vi "WVDIAL_Main.vi"() -> ()   [LabVIEW 2012]
uses:
  WVDIAL_GlobalVariables.vi
  TypeDefinitions.llb/TypeDef_LoopStagesMain.ctl
  TypeDefinitions.llb/TypeDef_ConfigureFIleTypes.ctl
  TypeDefinitions.llb/TypeDef_MainControlSystem.ctl
  TypeDefinitions.llb/TypeDef_ChildResponding.ctl
panel:
  out "Children Responding":T1[](array[typedef])
  out "LoopCounter":i32
  out "Permission Level":T3(ring)
  in  "User Comment":bool
  in  "Update Permissions":bool
  in  "Global Abort":bool
  in  "Tab Control":T4(tab)
  in  "Software Testing":bool
  in  "Template":bool
  in  "Operations":bool
  in  "Warmup":bool
  out "error IO":errorcluster
  out "SubPanelWidth":i32
  out "SubPanelHeight":i32
  out "What to Do":string
  out "QueueElement":string
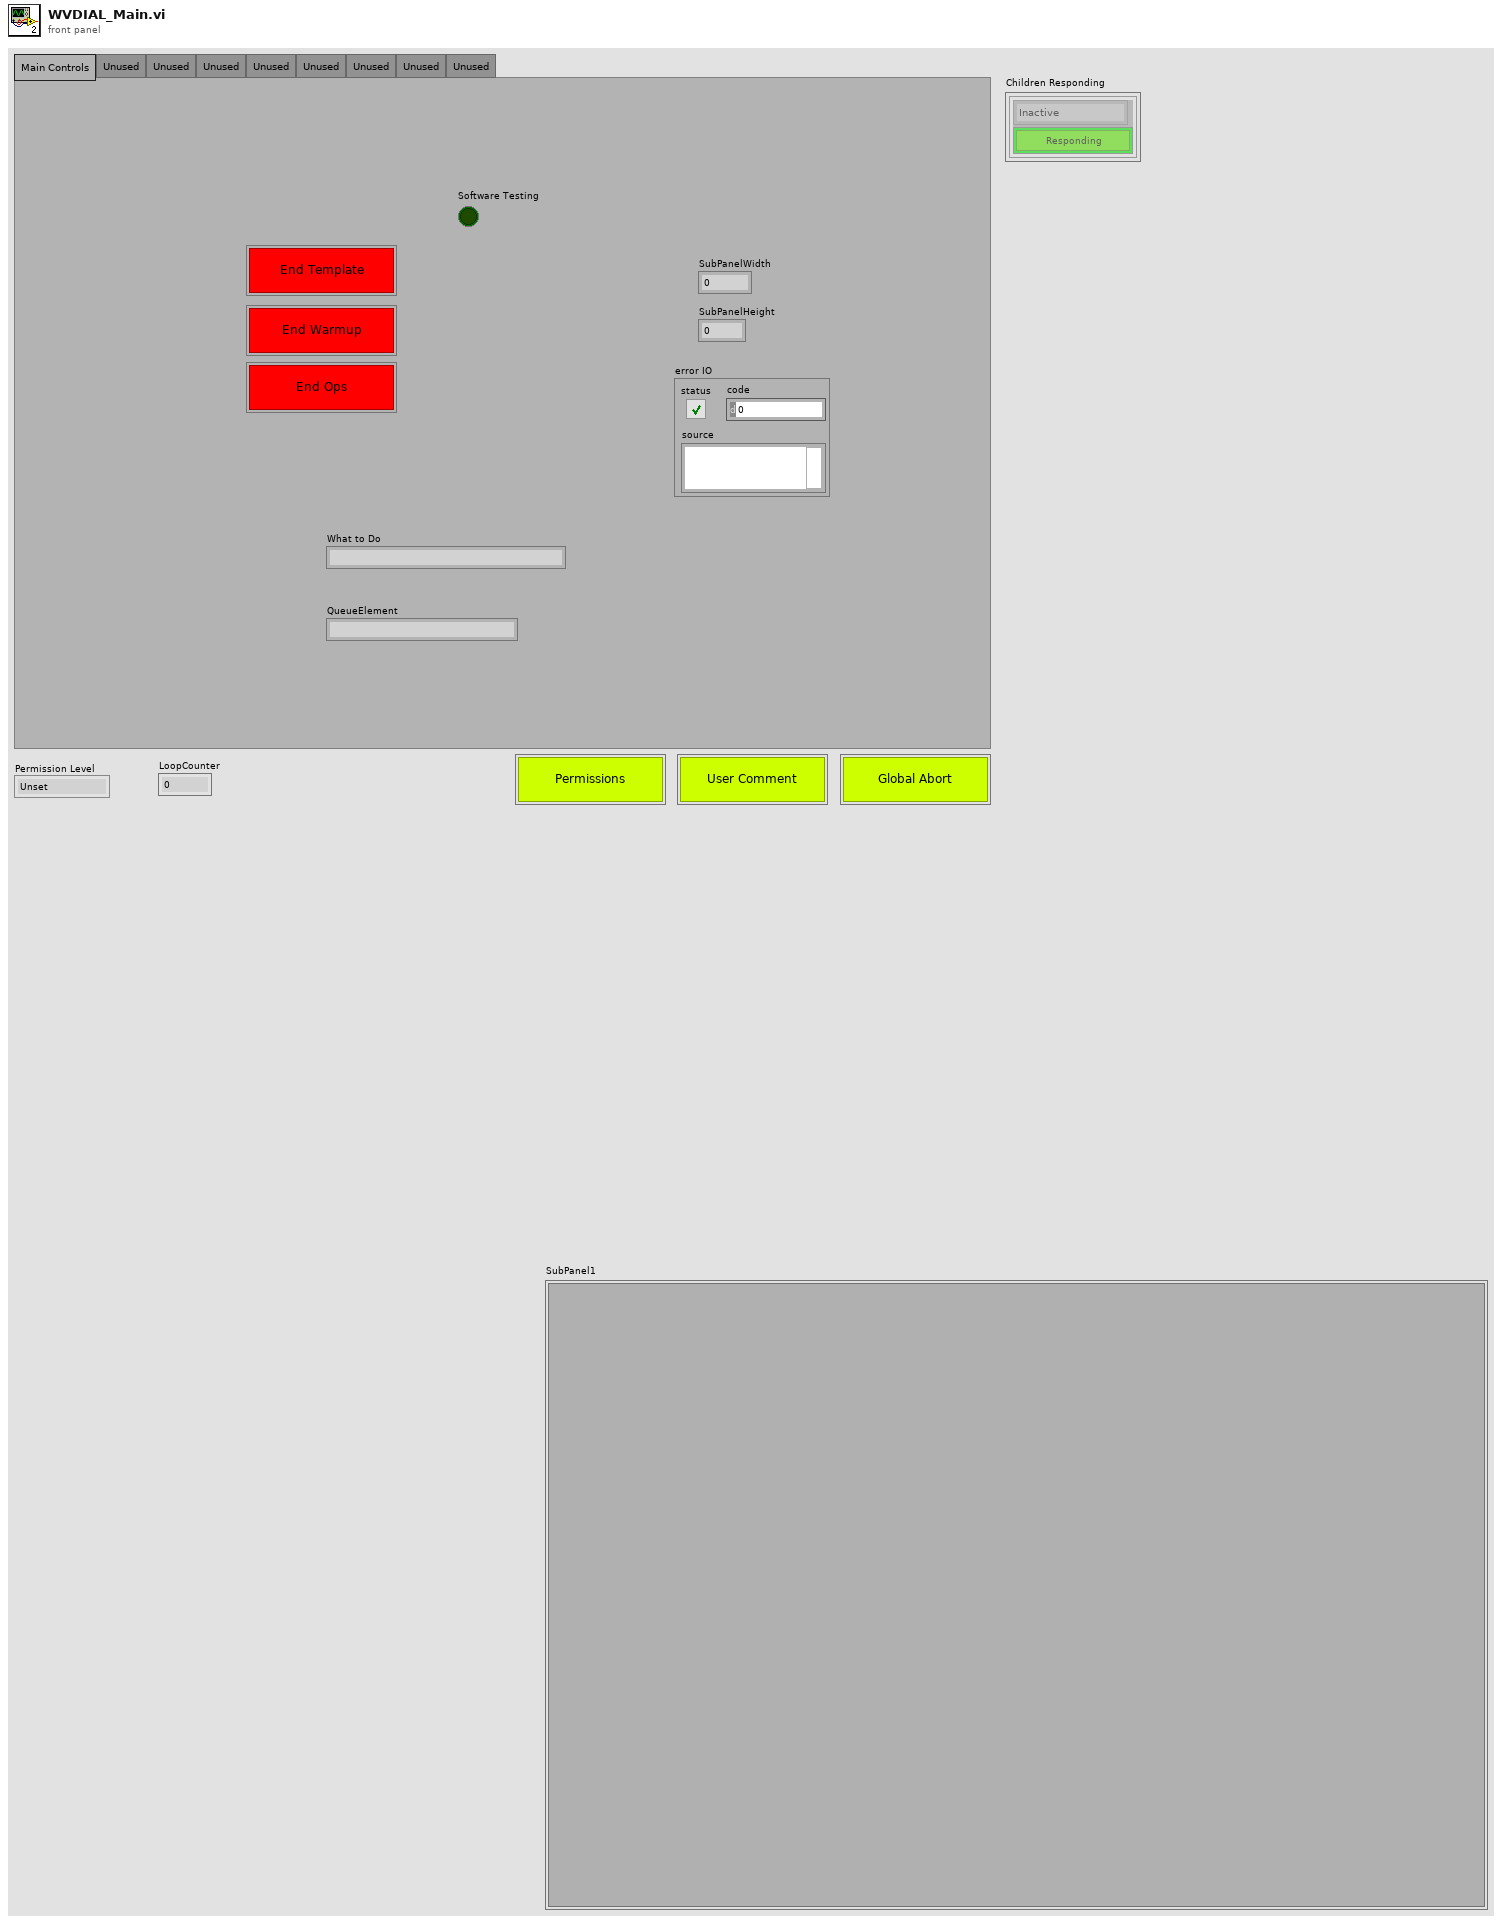
[diagram p1: front panel]
types:
  T1 = typedef "TypeDef_ChildResponding.ctl" = cluster{"MainControlSystems":T2, "Responding":bool}
  T2 = typedef "TypeDef_MainControlSystem.ctl" = enum16{"Inactive", "MCSControl", "MCSDisplay", "LaserControl", "LaserLocking", "WeatherStation", "DataDisplay", "Template"}
  T3 = enum16{"Unset", "Operator", "Administrator", "Full"}
  T4 = enum32{"Main Controls", "Inner Function 1", "Inner Function 2", "Inner Function 3", "Inner Function 4", "Inner Function 5", "Inner Function 6", "Inner Function 7", "Inner Function 8"}
  T5 = typedef "TypeDef_LoopStagesMain.ctl" = enum16{"Configure", "Initialize", "Idle", "ExitChildren", "Error Handler", "Exit"}
  T6 = typedef "TypeDef_ConfigureFIleTypes.ctl" = enum16{"Main", "OpsMain", "OpsTemplate", "OpsWarmup", "ChildHousekeeping", "ChildLaserLocking", "ChildMCS", "ChildMCSControl", "ChildPowerSwitches", "ChildQuantumComposer", "ChildTemplate", "ChildUPS", "ChildWeatherStation", "ChildPlotting", "TestingSwitches", "TestingWavemeter"}
  T7 = cluster{"MainControlSystems":T2, "Responding":bool}[]
  T8 = cluster{"Child Command Stop":bool, "Child Responding":bool, "MainControlSystems":T2, "LastReportTime":dbl, "Child Exiting":bool}[]
  T9 = enum32{"Page Enabled", "Page Disabled", "Page Disabled & Grayed"}
  T10 = cluster{"Child Command Stop":bool, "Child Responding":bool, "MainControlSystems":T2, "LastReportTime":dbl, "Child Exiting":bool}
  T11 = typedef "TypeDef_ChildReporting.ctl" = cluster{"Child Command Stop":bool, "Child Responding":bool, "MainControlSystems":T2, "LastReportTime":dbl, "Child Exiting":bool}
  T12 = enum32{"Bad", "Idle", "Run top level", "Running"}
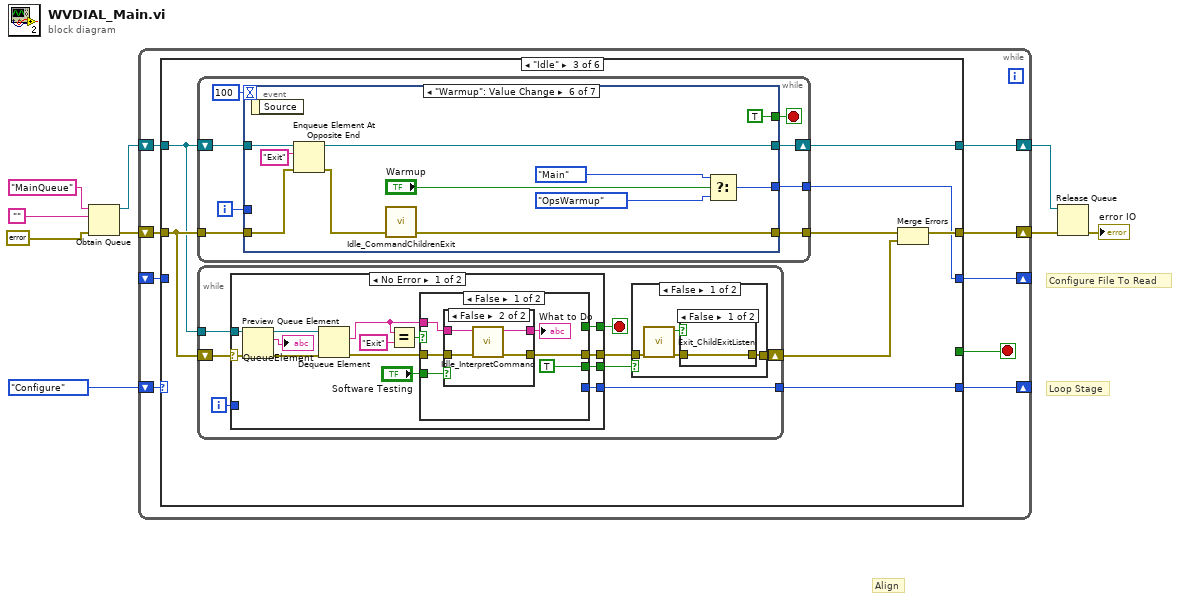
[diagram p0: block diagram]
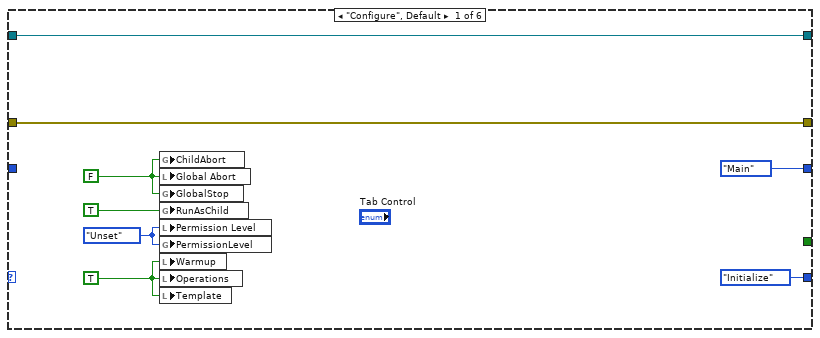
[diagram p2: hidden frame]
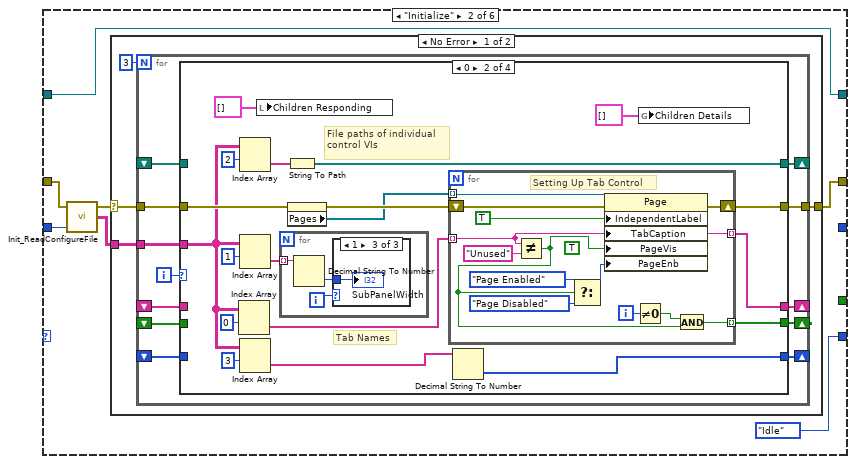
[diagram p3: hidden frame]
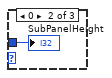
[diagram p6: hidden frame]
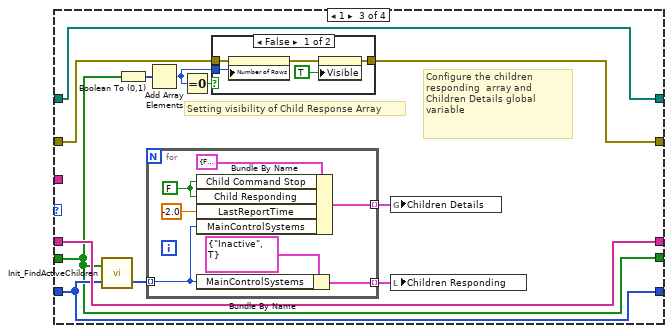
[diagram p7: hidden frame]
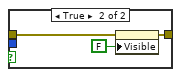
[diagram p8: hidden frame]
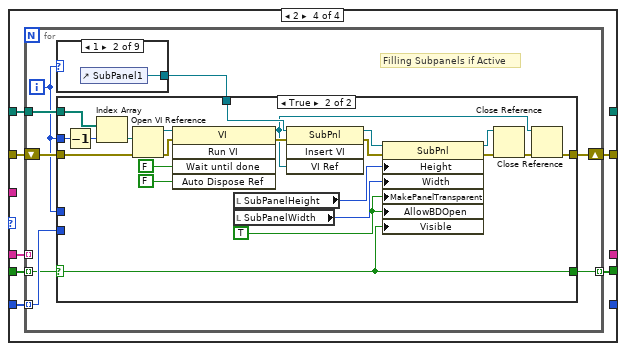
[diagram p9: hidden frame]
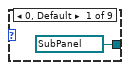
[diagram p11: hidden frame]
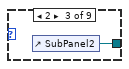
[diagram p12: hidden frame]
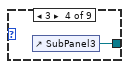
[diagram p13: hidden frame]
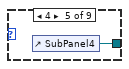
[diagram p14: hidden frame]
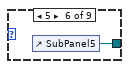
[diagram p15: hidden frame]
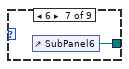
[diagram p16: hidden frame]
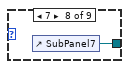
[diagram p17: hidden frame]
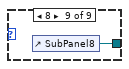
[diagram p18: hidden frame]
diagram:
  # "Align"
  # "Configure File To Read"
  # "Loop Stage"
  n1 = Obtain Queue(name (unnamed)="MainQueue", element data type="", error in (no error)=errorcluster {"status"=FALSE, "code"=0, "source"=""}) -> (queue out=w2:refnum<queue>, error out=w3:errorcluster)  [unwired: 2 in, 1 out]
  n2 = while {
    shift-right: [w14] -> w7
    shift-left: w3 -> [w15]
    shift-right: [w13] -> w8
    shift-left: w2 -> [w12]
    shift-right: [w17] -> _
    shift-left: TypeDef_LoopStagesMain."Configure" ("Enum") -> [w18]
    shift-right: [w11] -> _
    shift-left: _ -> [w10]
    stop <- w16 stop-if-true
    n3 = case shown="\"Idle\"" w18 {
      tunnel: [TypeDef_LoopStagesMain."Initialize" ("Enum") TypeDef_LoopStagesMain."Idle" ("Enum") w173 TypeDef_LoopStagesMain."Initialize" ("Enum") TypeDef_LoopStagesMain."Idle" ("Enum") TypeDef_LoopStagesMain."Exit" ("Enum")] -> w17
      tunnel: [_ _ _ _ _ TRUE] -> w16
      tunnel: [w23 w32 w170 w290 w319 w321] -> w14
      tunnel: w15 -> [w23 w30 w174 w291 w319 w325]
      tunnel: [w24 w31 w175 w294 w317 w327] -> w13
      tunnel: w12 -> [w24 w31 w169 w294 w317 w327]
      tunnel: [TypeDef_ConfigureFIleTypes."Main" ("MainControlSystems") _ w168 w292 _ _] -> w11
      tunnel: w10 -> [_ w27 _ w292 _ _]
      frame "Configure", Default {
        w20 = TRUE ("Warmup")
        w19 = T3."Unset" ("Permission Level")
        w21 = FALSE ("Global Stop")
        n4 = global write "WVDIAL_GlobalVariables.vi" "ChildAbort"(w21) -> ()
        n5 = local write "Global Abort"(w21) -> ()
        n6 = global write "WVDIAL_GlobalVariables.vi" "GlobalStop"(w21) -> ()
        n7 = global write "WVDIAL_GlobalVariables.vi" "RunAsChild"(TRUE ("RunAsChild")) -> ()
        n8 = local write "Permission Level"(w19) -> ()
        n9 = global write "WVDIAL_GlobalVariables.vi" "PermissionLevel"(w19) -> ()
        n10 = local write "Warmup"(w20) -> ()
        n11 = local write "Operations"(w20) -> ()
        n12 = local write "Template"(w20) -> ()
      }
      frame "Initialize" {
        n13 = call "Init_ReadConfigureFile.vi"("ConfigureFileType"=w27, "error in"=w30) -> ("Parsed List"=w28:string[][], "error out"=w29:errorcluster)  [unwired: 1 in, 1 out]
        n14 = case shown="No Error" w29 {
          selector: w29 -> [w36 w167]
          tunnel: [w37 w167] -> w32
          tunnel: w28 -> [w35 _]
          frame No Error {
            n15 = for {
              N: 3 -> [_]
              tunnel: [w49] -> w37
              tunnel: w36 -> [w40]
              tunnel: w35 -> [w47]
              shift-right: [w46] -> _
              shift-left: _ -> [w45]
              shift-right: [w44] -> _
              shift-left: _ -> [w43]
              shift-right: [w42] -> _
              shift-left: _ -> [w41]
              shift-right: [w39] -> _
              shift-left: _ -> [w38]
              i -> [w48]
              n16 = case shown="0" w48 {
                tunnel: [w53 w64 w100 w125] -> w49
                tunnel: w40 -> [w53 w63 w101 w121]
                tunnel: w47 -> [_ w59 _ _]
                tunnel: [w54 w69 w93 _] -> w46
                tunnel: w45 -> [w54 _ w93 w124]
                tunnel: [w52 w66 w97 _] -> w44
                tunnel: w43 -> [w52 _ w97 w123]
                tunnel: [w51 w65 w95 w120] -> w42
                tunnel: w41 -> [w51 _ w95 w122]
                tunnel: [w50 w57 w96 _] -> w39
                tunnel: w38 -> [w50 _ w96 w119]
                frame -1, Default {
                }
                frame 0 {
                  # "File paths of individual control VIs"
                  # "Tab Names"
                  n17 = Index Array(array=w59, index (row)=0) -> (element=w67:string[])  [unwired: 1 in]
                  n18 = Index Array(array=w59, index (row)=2) -> (element=w70:string[])  [unwired: 1 in]
                  n19 = Index Array(array=w59, index (row)=1) -> (element=w68:string[])  [unwired: 1 in]
                  n20 = Index Array(array=w59, index (row)=3) -> (element=w58:string[])  [unwired: 1 in]
                  n21 = local write "Children Responding"(T7 [] ("Children Responding")) -> ()
                  n22 = for {
                    tunnel: w68 -> [w88] mode=indexing
                    i -> [w89]
                    n23 = Decimal String To Number(string=w88) -> (number=w87:i32)  [unwired: 2 in, 1 out]
                    n24 = case shown="1" w89 {
                      tunnel: w87 -> [_ w90 w91]
                      frame -1, Default {
                      }
                      frame 0 {
                        "SubPanelHeight" <- w90
                      }
                      frame 1 {
                        "SubPanelWidth" <- w91
                      }
                    }
                  }
                  n25 = String To Path(string=w70) -> (path=w69:path[])
                  n26 = property on="Tab Control" class="TabCtl (strict)"(error in=w63) -> (error out=w62:errorcluster, "Pages"=w61:refnum<vi>[])  [unwired: 1 in, 1 out]
                  n27 = for {
                    tunnel: w67 -> [w80] mode=indexing
                    tunnel: w61 -> [w83] mode=indexing
                    shift-right: [w81] -> w64
                    shift-left: w62 -> [w82]
                    tunnel: [w80] -> w66 mode=indexing
                    tunnel: [w77] -> w65 mode=indexing
                    i -> [w78]
                    (unwired) TRUE ("Page Visible")
                    # "Setting Up Tab Control"
                    n28 = Not Equal?(x=w80, y="Unused") -> (x != y?=w76:bool)
                    n29 = Select(t=T9."Page Enabled" ("Page Enabled State"), s=w76, f=T9."Page Disabled" ("Page Enabled State")) -> (s? t:f=w74:T9)
                    n30 = property class="Page"(reference=w83, error in=w82, "IndependentLabel"=TRUE ("Independent Label"), "TabCaption"=w80, "PageVis"=w76, "PageEnb"=w74) -> (error out=w81:errorcluster)  [unwired: 1 out]
                    n31 = Not Equal To 0?(x=w78) -> (x != 0?=w79:bool)
                    n32 = And(x=w79, y=w76) -> (x .and. y?=w77:bool)
                  }
                  n33 = Decimal String To Number(string=w58) -> (number=w57:i32[])  [unwired: 2 in, 1 out]
                  n34 = global write "WVDIAL_GlobalVariables.vi" "Children Details"(T8 []) -> ()
                }
                frame 1 {
                  # "Setting visibility of Child Response Array"
                  # "Configure the children responding  array and Children Details global variable"
                  n35 = call "Init_FindActiveChildren.vi"("ChannelType"=w96, "ChannelOn"=w95) -> ("ActiveTypes"=w94:i32[])  [unwired: 1 out]
                  n36 = Boolean To (0,1)(Boolean=w95) -> (0, 1=w103:i16[])
                  n37 = for {
                    tunnel: [w118] -> w102 mode=indexing
                    tunnel: w94 -> [w114] mode=indexing
                    tunnel: [w117] -> w92 mode=indexing
                    w116 = FALSE
                    n38 = Bundle By Name(cluster=T10 {"Child Command Stop"=FALSE, "Child Responding"=FALSE, "MainControlSystems"=enum."Inactive", "LastReportTime"=0.0, "Child Exiting"=FALSE} ("Child Details"), "Child Command Stop"=w116, "Child Responding"=w116, "LastReportTime"=-2.0, "MainControlSystems"=w114) -> (w117:T10)
                    n39 = Bundle By Name(cluster=T1 {"MainControlSystems"=enum."Inactive", "Responding"=TRUE} ("ChildResponse"), "MainControlSystems"=w114) -> (w118:T1)
                  }
                  n40 = Add Array Elements(numeric array=w103) -> (sum=w99:i16)
                  n41 = Equal To 0?(x=w99) -> (x = 0?=w98:bool)
                  n42 = case shown="False" w98 {
                    tunnel: w101 -> [w108 w111]
                    tunnel: [w105 w110] -> w100
                    tunnel: w99 -> [w107 _]
                    frame False {
                      n43 = property on="Children Responding" class="Arr (strict)"(error in=w108, "Number of Rows"=w107) -> (error out=w106:errorcluster)  [unwired: 1 in, 1 out]
                      n44 = property on="Children Responding" class="Arr (strict)"(error in=w106, "Visible"=TRUE) -> (error out=w105:errorcluster)  [unwired: 1 in, 1 out]
                    }
                    frame True {
                      n45 = property on="Children Responding" class="Arr (strict)"(error in=w111, "Visible"=FALSE) -> (error out=w110:errorcluster)  [unwired: 1 in, 1 out]
                    }
                  }
                  n46 = global write "WVDIAL_GlobalVariables.vi" "Children Details"(w92) -> ()
                  n47 = local write "Children Responding"(w102) -> ()
                }
                frame 2 {
                  n48 = for {
                    shift-right: [w132] -> w125
                    shift-left: w121 -> [w133]
                    tunnel: w123 -> [_] mode=indexing
                    tunnel: w124 -> [w131]
                    tunnel: w122 -> [w126] mode=indexing
                    tunnel: [w129] -> w120 mode=indexing
                    tunnel: w119 -> [w128] mode=indexing
                    i -> [w127]
                    # "Filling Subpanels if Active"
                    n49 = case shown="1" w127 {
                      tunnel: [refnum<vi> refnum ("SubPanel1") w159 w160 w161 w162 w163 w164 w165 w166] -> w130
                      frame 0, Default {
                      }
                      frame 1 {
                        n50 = control-ref of="SubPanel1"() -> (w159:refnum<vi>)
                      }
                      frame 2 {
                        n51 = control-ref of="SubPanel2"() -> (w160:refnum<vi>)
                      }
                      frame 3 {
                        n52 = control-ref of="SubPanel3"() -> (w161:refnum<vi>)
                      }
                      frame 4 {
                        n53 = control-ref of="SubPanel4"() -> (w162:refnum<vi>)
                      }
                      frame 5 {
                        n54 = control-ref of="SubPanel5"() -> (w163:refnum<vi>)
                      }
                      frame 6 {
                        n55 = control-ref of="SubPanel6"() -> (w164:refnum<vi>)
                      }
                      frame 7 {
                        n56 = control-ref of="SubPanel7"() -> (w165:refnum<vi>)
                      }
                      frame 8 {
                        n57 = control-ref of="SubPanel8"() -> (w166:refnum<vi>)
                      }
                    }
                    n58 = case shown="True" w126 {
                      selector: w126 -> [w134 w145]
                      tunnel: w133 -> [w135 w157]
                      tunnel: [w135 w138] -> w132
                      tunnel: w131 -> [_ w156]
                      tunnel: w127 -> [_ w144]
                      tunnel: w130 -> [_ w155]
                      tunnel: [w134 w145] -> w129
                      tunnel: w128 -> [_ _]
                      tunnel: w127 -> [_ _]
                      frame False {
                      }
                      frame True {
                        w146 = TRUE ("Allow User to Open Diagram")
                        n59 = Decrement(x=w144) -> (x-1=w143:i32)
                        n60 = Index Array(array=w156, index=w143) -> (element=w154:path)
                        n61 = Open VI Reference(vi path=w154, error in (no error)=w157) -> (vi reference=w153:refnum<vi>, error out=w152:errorcluster)  [unwired: 4 in]
                        n62 = invoke class="VI" method="Run VI"(reference=w153, error in=w152, "Wait until done"=FALSE ("Wait Until Done"), "Auto Dispose Ref"=FALSE ("Auto Dispose Reference")) -> (reference out=w136:refnum<vi>, error out=w150:errorcluster)  [unwired: 1 in, 3 out]
                        n63 = local read "SubPanelHeight"() -> (w148:i32)
                        n64 = local read "SubPanelWidth"() -> (w147:i32)
                        n65 = invoke on="Invoke Node" class="SubPnl" method="Insert VI"(reference=w155, error in=w150, "VI Ref"=w136) -> (reference out=w137:refnum<vi>, error out=w149:errorcluster)  [unwired: 1 in, 2 out]
                        n66 = property on="Property Node" class="SubPnl"(reference=w137, error in=w149, "Height"=w148, "Width"=w147, "MakePanelTransparent"=w146, "AllowBDOpen"=w146, "Visible"=w145) -> (reference out=w140:refnum<vi>, error out=w141:errorcluster)
                        n67 = Close Reference(reference=w140, error in (no error)=w141) -> (error out=w139:errorcluster)
                        n68 = Close Reference(reference=w136, error in (no error)=w139) -> (error out=w138:errorcluster)
                      }
                    }
                  }
                }
              }
            }
          }
          frame Error {
          }
        }
      }
      frame "Idle" {
        n69 = while {
          tunnel: w174 -> [w232]
          shift-right: [w227] -> w175
          shift-left: w169 -> [w228]
          tunnel: [w226] -> w171
          tunnel: [w225] -> w168
          i -> [w229]
          stop <- w230 stop-if-true
          n70 = event shown="[5] \"Warmup\": Value Change" {
            selector: _ -> [_ _ _ _ _ _ _]
            dyn-events: _ -> [_ _ _ _ _ _ _]
            timeout: 100 -> [_ _ _ _ _ _ _]
            tunnel: w232 -> [w239 w244 w249 w254 w262 w273 w284]
            tunnel: [_ "Global Abort" _ _ TRUE ("Global Abort") TRUE ("Global Abort") TRUE ("Global Abort")] -> w230
            tunnel: w229 -> [w238 _ _ _ _ _ _]
            tunnel: w228 -> [w237 w242 w247 w252 w264 w275 w286]
            tunnel: [w237 w241 w246 w251 w263 w274 w285] -> w227
            tunnel: [w239 w243 w248 w253 w256 w268 w279] -> w226
            tunnel: [_ _ _ _ w266 w277 w288] -> w225
            event Timeout {
              n71 = event-data() -> ()  [unwired: 1 in, 1 out]
              n72 = global read "WVDIAL_GlobalVariables.vi" "PermissionLevel"() -> (→"Permission Level":i32)
              n73 = local read "Children Responding"() -> (w234:T1[])
              n74 = call "Idle_MainIdleProcess.vi"("ChildrenResponding"=w234) -> ("ChildrenDetailsUpdated"=w236:T11[], "ChildrenResponding"=→"Children Responding":T1[])  [unwired: 1 in]
              n75 = global write "WVDIAL_GlobalVariables.vi" "Children Details"(w236) -> ()
              "LoopCounter" <- w238
            }
            event "Global Abort": Value Change {
              n76 = event-data() -> ()  [unwired: 1 in, 1 out]
              n77 = Enqueue Element(queue=w242, element="Exit", error in (no error)=w244) -> (queue out=w241:refnum<queue>, error out=w243:errorcluster)  [unwired: 1 in, 1 out]
              n78 = global write "WVDIAL_GlobalVariables.vi" "GlobalStop"("Global Abort") -> ()
            }
            event "Update Permissions": Value Change {
              n79 = event-data() -> ()  [unwired: 1 in, 1 out]
              n80 = Enqueue Element(queue=w247, element="System_OpenPermissionsVI", error in (no error)=w249) -> (queue out=w246:refnum<queue>, error out=w248:errorcluster)  [unwired: 1 in, 1 out]
            }
            event "User Comment": Value Change {
              n81 = event-data() -> ()  [unwired: 1 in, 1 out]
              n82 = Enqueue Element(queue=w252, element="System_OpenUserCommentVI", error in (no error)=w254) -> (queue out=w251:refnum<queue>, error out=w253:errorcluster)  [unwired: 1 in, 1 out]
            }
            event "Template": Value Change {
              n83 = event-data() -> ()  [unwired: 1 in, 1 out]
              n84 = Enqueue Element At Opposite End(queue=w264, element="Exit", error in (no error)=w262) -> (queue out=w263:refnum<queue>, error out=w257:errorcluster)  [unwired: 1 in, 1 out]
              n85 = call "Idle_CommandChildrenExit.vi"("ErrorIn"=w257) -> ("ErrorOut"=w256:errorcluster)  [unwired: 4 in]
              n86 = Select(t=TypeDef_ConfigureFIleTypes."Main" ("MainControlSystems"), s="Template", f=TypeDef_ConfigureFIleTypes."OpsTemplate" ("MainControlSystems")) -> (s? t:f=w266:T6)
            }
            event "Warmup": Value Change {
              n87 = event-data() -> ()  [unwired: 1 in, 1 out]
              n88 = Enqueue Element At Opposite End(queue=w275, element="Exit", error in (no error)=w273) -> (queue out=w274:refnum<queue>, error out=w269:errorcluster)  [unwired: 1 in, 1 out]
              n89 = call "Idle_CommandChildrenExit.vi"("ErrorIn"=w269) -> ("ErrorOut"=w268:errorcluster)  [unwired: 4 in]
              n90 = Select(t=TypeDef_ConfigureFIleTypes."Main" ("MainControlSystems"), s="Warmup", f=TypeDef_ConfigureFIleTypes."OpsWarmup" ("MainControlSystems")) -> (s? t:f=w277:T6)
            }
            event "Operations": Value Change {
              n91 = event-data() -> ()  [unwired: 1 in, 1 out]
              n92 = Enqueue Element At Opposite End(queue=w286, element="Exit", error in (no error)=w284) -> (queue out=w285:refnum<queue>, error out=w280:errorcluster)  [unwired: 1 in, 1 out]
              n93 = call "Idle_CommandChildrenExit.vi"("ErrorIn"=w280) -> ("ErrorOut"=w279:errorcluster)  [unwired: 4 in]
              n94 = Select(t=TypeDef_ConfigureFIleTypes."Main" ("MainControlSystems"), s="Operations", f=TypeDef_ConfigureFIleTypes."OpsMain" ("MainControlSystems")) -> (s? t:f=w288:T6)
            }
          }
        }
        n95 = while {
          tunnel: w169 -> [w182]
          tunnel: [w181] -> w173
          shift-right: [w178] -> w172
          shift-left: w174 -> [w183]
          i -> [w180]
          stop <- w177 stop-if-true
          n96 = case shown="No Error" w183 {
            selector: w183 -> [w202 w224]
            tunnel: w182 -> [w201 _]
            tunnel: [w195 _] -> w177
            tunnel: [w194 _] -> w181
            tunnel: [w193 w224] -> w179
            tunnel: w180 -> [_ _]
            tunnel: [w192 TRUE ("GlobalStop")] -> w176
            frame No Error {
              n97 = Preview Queue Element(queue=w201, error in (no error)=w202) -> (queue out=w204:refnum<queue>, element=→"QueueElement":string, error out=w203:errorcluster)  [unwired: 1 in, 1 out]
              n98 = Dequeue Element(queue=w204, error in (no error)=w203) -> (element=w196:string, error out=w198:errorcluster)  [unwired: 1 in, 2 out]
              n99 = Equal?(x=w196, y="Exit") -> (x = y?=w197:bool)
              n100 = case shown="False" w197 {
                tunnel: w198 -> [w209 w218]
                tunnel: w196 -> [w206 _]
                tunnel: [_ TRUE] -> w195
                tunnel: [_ w219] -> w194
                tunnel: [w208 w218] -> w193
                tunnel: [TRUE ("GlobalStop") w217] -> w192
                tunnel: "Software Testing" -> [w210 _]
                frame False {
                  n101 = case shown="False" w210 {
                    tunnel: w209 -> [w212 w216]
                    tunnel: [w212 w215] -> w208
                    tunnel: w206 -> [_ w214]
                    tunnel: ["" w213] -> w205
                    frame True {
                    }
                    frame False {
                      n102 = call "Idle_InterpretCommand.vi"("error in"=w216, "Input Command"=w214) -> ("error out"=w215:errorcluster, "What to Do"=w213:string)  [unwired: 8 in]
                    }
                  }
                  "What to Do" <- w205
                }
                frame True {
                  n103 = global read "WVDIAL_GlobalVariables.vi" "GlobalStop"() -> (w217:bool)
                  n104 = Select(t=TypeDef_LoopStagesMain."Exit" ("Enum"), s=w217, f=TypeDef_LoopStagesMain."ExitChildren" ("Enum")) -> (s? t:f=w219:T5)
                }
              }
            }
            frame Error {
            }
          }
          n105 = case shown="False" w176 {
            tunnel: w179 -> [w187 w190]
            tunnel: [w185 w190] -> w178
            frame False {
              n106 = call "Exit_ChildExitListen.vi"("ErrorIn"=w187) -> ("ErrorOut"=w186:errorcluster, "TimedOut"=w184:bool)  [unwired: 9 in]
              n107 = case shown="False" w184 {
                tunnel: w186 -> [w188 w189]
                tunnel: [w188 w189] -> w185
                frame False {
                }
                frame True {
                }
              }
            }
            frame True {
            }
          }
        }
        n108 = Merge Errors(w171, w172) -> (w170:errorcluster)
      }
      frame "ExitChildren" {
        n109 = for {
          N: 9 -> [_]
          shift-right: [w297] -> w290
          shift-left: w291 -> [w305]
          tunnel: [w295] -> _ mode=indexing
          i -> [w307]
          n110 = case shown="1" w307 {
            tunnel: [refnum<vi> refnum ("SubPanel1") w309 w310 w311 w312 w313 w314 w315 w316] -> w306
            frame 0, Default {
            }
            frame 1 {
              n111 = control-ref of="SubPanel1"() -> (w309:refnum<vi>)
            }
            frame 2 {
              n112 = control-ref of="SubPanel2"() -> (w310:refnum<vi>)
            }
            frame 3 {
              n113 = control-ref of="SubPanel3"() -> (w311:refnum<vi>)
            }
            frame 4 {
              n114 = control-ref of="SubPanel4"() -> (w312:refnum<vi>)
            }
            frame 5 {
              n115 = control-ref of="SubPanel5"() -> (w313:refnum<vi>)
            }
            frame 6 {
              n116 = control-ref of="SubPanel6"() -> (w314:refnum<vi>)
            }
            frame 7 {
              n117 = control-ref of="SubPanel7"() -> (w315:refnum<vi>)
            }
            frame 8 {
              n118 = control-ref of="SubPanel8"() -> (w316:refnum<vi>)
            }
          }
          n119 = property class="SubPnl"(reference=w306, error in=w305) -> (reference out=w296:refnum<vi>, error out=w300:errorcluster, "InsertedVI"=w299:refnum<vi>)
          n120 = property class="VI"(reference=w299, error in=w300) -> (reference out=w301:refnum<vi>, error out=w302:errorcluster, "Exec.State"=w295:T12)
          n121 = invoke on="Invoke Node" class="VI" method="FP.Close"(reference=w301, error in=w302) -> (reference out=w303:refnum<vi>, error out=w304:errorcluster)  [unwired: 1 in, 1 out]
          n122 = Close Reference(reference=w303, error in (no error)=w304) -> (error out=w298:errorcluster)
          n123 = Close Reference(reference=w296, error in (no error)=w298) -> (error out=w297:errorcluster)
        }
      }
      frame "Error Handler" {
      }
      frame "Exit" {
        n124 = property on="Tab Control" class="TabCtl (strict)"(error in=w325) -> (error out=w324:errorcluster, "Pages"=w323:refnum<vi>[])  [unwired: 1 in, 1 out]
        n125 = global write "WVDIAL_GlobalVariables.vi" "RunAsChild"(FALSE ("RunAsChild")) -> ()
        n126 = local write "Permission Level"(T3."Unset" ("Permission Level")) -> ()
        n127 = for {
          shift-right: [w332] -> w322
          shift-left: w324 -> [w334]
          tunnel: w323 -> [w333] mode=indexing
          n128 = property class="Page"(reference=w333, error in=w334, "PageVis"=TRUE ("Page Visible")) -> (error out=w332:errorcluster)  [unwired: 1 out]
        }
        n129 = property on="Children Responding" class="Arr (strict)"(error in=w322, "Visible"=TRUE) -> (error out=w321:errorcluster)  [unwired: 1 in, 1 out]
      }
    }
  }
  n130 = Release Queue(queue=w8, error in (no error)=w7) -> (error out=→"error IO":errorcluster)  [unwired: 1 in, 2 out]
